vi "SA_PRESET.vi"(8 "error in":errorcluster {"code" format="%.0x"}, 11 "Session In":refnum<visa-resource-name>="TCPIP0::K-N90X0A-00005.local::hislip0::INSTR") -> (0 "error out":errorcluster {"code" format="%.0x"}, 3 "Session Out":refnum<visa-resource-name>)   [LabVIEW 2018]
doc: "Restore Input/Output Defaults\nThis selection causes the group of settings and data associated with the\nInput/Output key to be a reset to their default values. In addition, when a Source is\ninstalled, licensed and selected, Restore Input/Output defaults will initiate a Source\nPreset.\n Spectrum Analyzer Mode Reference\nInput/Output Functions\nInput/Output\nThis level of Restore System Defaults does not affect any other system settings or\nmode settings and does not cause a mode switch. All the features described in this\nsection are reset using this key, including Input Corrections and Data (described in\nthe Corrections section)."
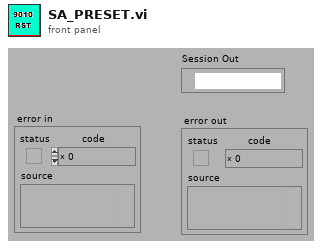
[diagram p1: front panel]
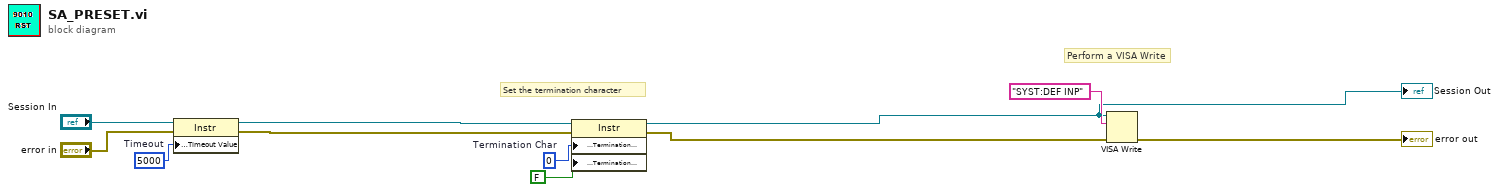
[diagram p0: block diagram]
diagram:
  w6 = u8 0  # Termination Char
  w11 = u32 5000  # Timeout
  # "Perform a VISA Write"
  # "Set the termination character"
  n1 = property class="Instr"(reference="Session In", error in="error in", "General Settings:Timeout Value"=w11) -> (reference out=w5:refnum<visa-resource-name>, error out=w8:errorcluster)
  n2 = property class="Instr"(reference=w5, error in=w8, "Message Based Settings:Termination Character"=w6, "Message Based Settings:Termination Character Enable"=FALSE ("enable")) -> (reference out=w1:refnum<visa-resource-name>, error out=w7:errorcluster)
  "Session Out" <- w1
  n3 = VISA Write(VISA resource name=w1, write buffer="SYST:DEF INP" ("StaticText"), error in (no error)=w7) -> (error out=→"error out":errorcluster)  [unwired: 2 out]
